vi "getCurrent.vi"(8 "error in (no error)":errorcluster, 10 "baseObject in":refnum<class "IBaseObject.lvclass">, 11 "IIterator in":refnum<class "IIterator.lvclass">) -> (0 "error out":errorcluster, 2 "baseObject out":refnum<class "IBaseObject.lvclass">, 3 "IIterator out":refnum<class "IIterator.lvclass">)   [LabVIEW 2022 SP3, in "openDAQ.lvlib" / "IBaseObject.lvlib" / "IIterator.lvlib" / "IIterator.lvclass"]
uses:
  <instrlib>/openDAQ/Public/Classes/IIterator/IIterator.lvclass
  C:/Program Files (x86)/National Instruments/LabVIEW 2022/instr.lib/openDAQ/Public/Classes/IBaseObject/IBaseObject.lvclass
  <instrlib>/openDAQ/Public/Classes/IBaseObject/IBaseObject.lvclass
  <instrlib>/openDAQ/Public/Classes/IBaseObject/IBaseObject.lvclass/IBaseObject.ctl
  <instrlib>/openDAQ/Public/Classes/IBaseObject/Accessor/Read reference.vi
  <instrlib>/openDAQ/Public/Classes/IBaseObject/Accessor/Write reference.vi
  <instrlib>/openDAQ/Binaries/Windows/x86/copendaq32.dll
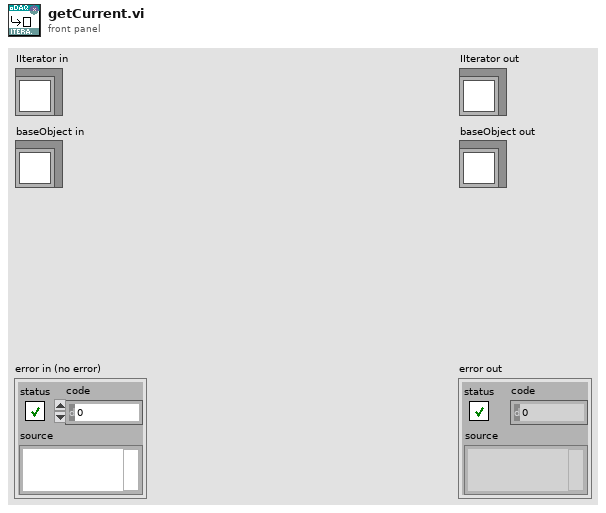
[diagram p1: front panel]
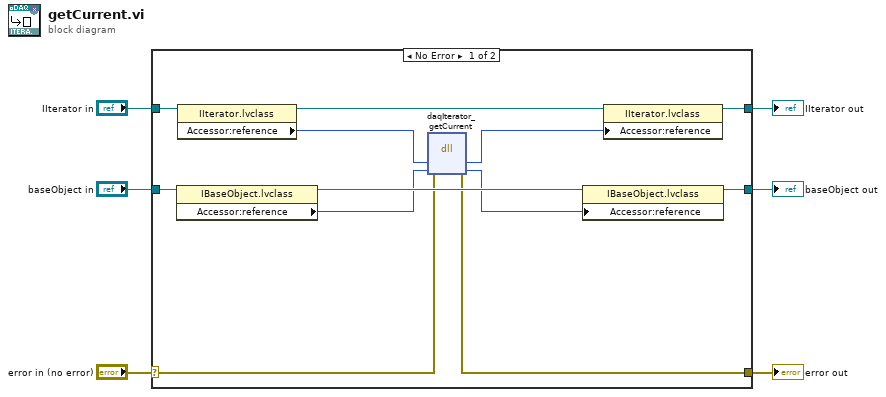
[diagram p0: block diagram]
diagram:
  n1 = case shown="No Error" "error in (no error)" {
    selector: "error in (no error)" -> [w9 w21]
    tunnel: [w8 w21] -> w5
    tunnel: [w15 w20] -> w4
    tunnel: "IIterator in" -> [w17 w20]
    tunnel: "baseObject in" -> [w12 w19]
    tunnel: [w7 w19] -> w1
    frame No Error {
      n2 = property class="IBaseObject.lvclass"(reference=w12) -> (reference out=w18:refnum<class "IBaseObject.lvclass">, "Accessor:reference"=w11:i64)  [unwired: 1 in, 1 out]
      n3 = property class="IIterator.lvclass"(reference=w17) -> (reference out=w16:refnum<class "IIterator.lvclass">, "Accessor:reference"=w14:i64)  [unwired: 1 in, 1 out]
      n4 = dll-call lib="C:/Program Files (x86)/National Instruments/LabVIEW 2022/instr.lib/openDAQ/Binaries/Windows/x86/copendaq*.*" fn="daqIterator_getCurrent"(error in=w9, "iterator"=w14, "obj"=w11) -> (error out=w8:errorcluster, "iterator"=w13:i64, "obj"=w10:i64)  [unwired: 3 in, 1 out]
      n5 = property class="IBaseObject.lvclass"(reference=w18, "Accessor:reference"=w10) -> (reference out=w7:refnum<class "IBaseObject.lvclass">)  [unwired: 1 in, 1 out]
      n6 = property class="IIterator.lvclass"(reference=w16, "Accessor:reference"=w13) -> (reference out=w15:refnum<class "IIterator.lvclass">)  [unwired: 1 in, 1 out]
    }
    frame Error {
    }
  }
  "error out" <- w5
  "IIterator out" <- w4
  "baseObject out" <- w1
